vi "Constants.vi"() -> (1 "String Delimeter":string)   [LabVIEW 2017, in "XTree.xctl"]
doc: "Serves as storage for project-wide constants."
uses:
  <vilib>/addons/_NIFileIO/XTree/XTree.xctl
panel:
  # "This VI serves as storage for constants used throughout the XControl"
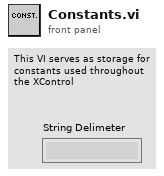
[diagram p1: front panel]
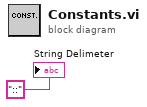
[diagram p0: block diagram]
diagram:
  "String Delimeter" <- "::" ("String Delimeter")
